vi "Log File Handler.vi"(9 "Event data":string, 10 "Event":string) -> ()   [LabVIEW 2025]
uses:
  <vilib>/Utility/file.llb/Write Delimited Spreadsheet (string).vi
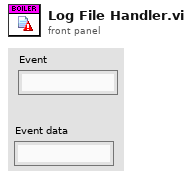
[diagram p1: front panel]
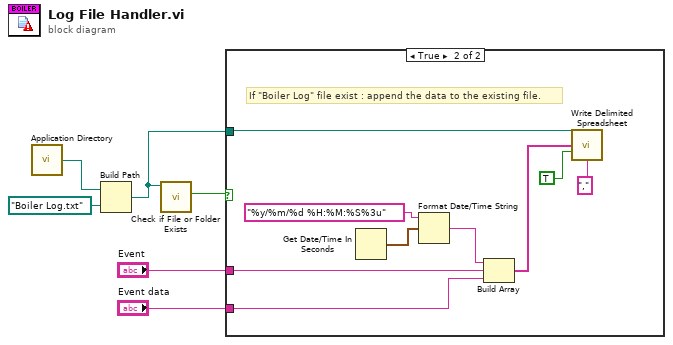
[diagram p0: block diagram]
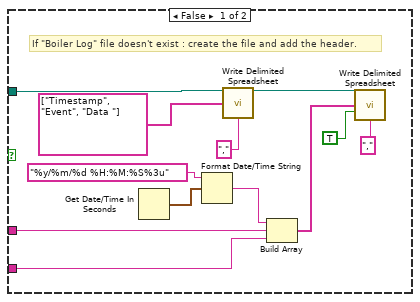
[diagram p2: hidden frame]
diagram:
  n1 = call <vilib>:"Application Directory.vi"() -> ("Application Directory"=w6:path)
  n2 = Build Path(base path=w6, name or relative path=path "Boiler Log.txt") -> (appended path=w3:path)
  n3 = call <vilib>:"Check if File or Folder Exists.vi"("path"=w3) -> ("file or folder exists?"=w4:bool)  [unwired: 8 in, 2 out]
  n4 = case shown="True" w4 {
    tunnel: w3 -> [w16 w19]
    tunnel: "Event" -> [w12 w24]
    tunnel: "Event data" -> [w11 w23]
    frame False {
      # "If \"Boiler Log\" file doesn't exist : create the file and add the header."
      n5 = Get Date/Time In Seconds() -> (seconds since 1Jan1904=w15:timestamp)
      n6 = Format Date/Time String(time format string (%c)="%y/%m/%d %H:%M:%S%3u", seconds (now)=w15) -> (date/time string=w13:string)  [unwired: 1 in]
      n7 = call-poly <vilib>:"Write Delimited Spreadsheet.vi"("file path (dialog if empty)"=w16, "1D data"=string[] ["Timestamp", "Event", "Data "], "delimiter (\\t)"="," ("delimiter (\\t)")) -> ("new file path (Not A Path if cancelled)"=w10:path)  [unwired: 11 in, 1 out]
      n8 = Build Array(w13, w12, w11) -> (w9:string[])
      n9 = call-poly <vilib>:"Write Delimited Spreadsheet.vi"("file path (dialog if empty)"=w10, "1D data"=w9, "append to file? (new file:F)"=TRUE, "delimiter (\\t)"="," ("delimiter (\\t)")) -> ()  [unwired: 10 in, 2 out]
    }
    frame True {
      # "If \"Boiler Log\" file exist : append the data to the existing file."
      n10 = Get Date/Time In Seconds() -> (seconds since 1Jan1904=w27:timestamp)
      n11 = Format Date/Time String(time format string (%c)="%y/%m/%d %H:%M:%S%3u", seconds (now)=w27) -> (date/time string=w25:string)  [unwired: 1 in]
      n12 = Build Array(w25, w24, w23) -> (w22:string[])
      n13 = call-poly <vilib>:"Write Delimited Spreadsheet.vi"("file path (dialog if empty)"=w19, "1D data"=w22, "append to file? (new file:F)"=TRUE, "delimiter (\\t)"="," ("delimiter (\\t)")) -> ()  [unwired: 10 in, 2 out]
    }
  }
